vi "C-726.1CD (Piezo).vi"(8 "error in":errorcluster, 11 "System no.":i32=1 min=1 max=4 step=1) -> (0 "error out":errorcluster, 2 "Conn. Axis":string[](array[string]), 3 "C-726.1CD":dbl[](array[numeric]) format="%.6f", 5 "Identification 2":string)   [LabVIEW 2011]
panel:
  in  "stop":bool
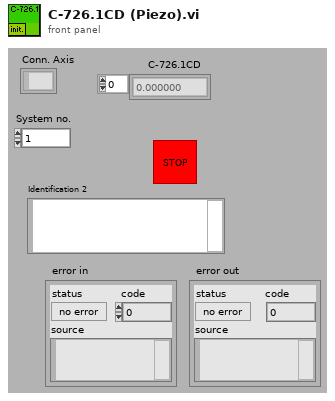
[diagram p1: front panel]
types:
  T1 = cluster{"Host address/name":string, "Port":i32, "Board":i32, "TCP/IP Search?":bool}
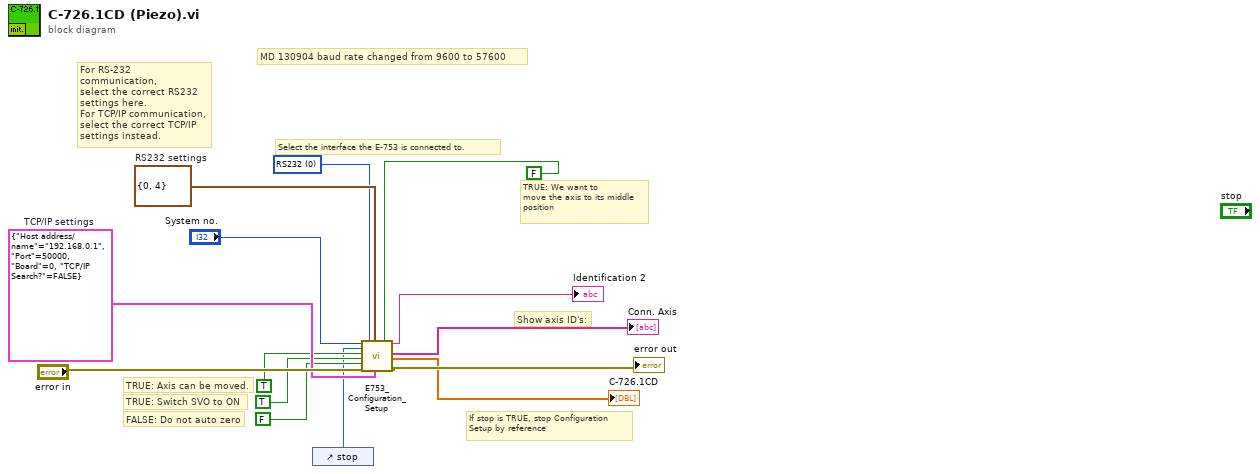
[diagram p0: block diagram]
diagram:
  w10 = cluster{"Portnumber":i32, "Baudrate":u16} {"Portnumber"=0, "Baudrate"=4}  # RS232 settings
  w11 = T1 {"Host address/name"="192.168.0.1", "Port"=50000, "Board"=0, "TCP/IP Search?"=FALSE}  # TCP/IP settings
  w8 = u16 0 items=["RS232", "TCP/IP"] ("Interface")
  # "MD 130904 baud rate changed from 9600 to 57600"
  # "TRUE: We want to\nmove the axis to its middle\nposition"
  # "FALSE: Do not auto zero"
  # "TRUE: Switch SVO to ON"
  # "If stop is TRUE, stop Configuration\nSetup by reference"
  # "For RS-232 communication,\nselect the correct RS232\nsettings here.\nFor TCP/IP communication, \nselect the correct TCP/IP\nsettings instead."
  # "Select the interface the E-753 is connected to."
  # "Show axis ID's:"
  # "TRUE: Axis can be moved."
  n1 = control-ref of="stop"() -> (w1:refnum<vi>)
  n2 = call "E753_Configuration_Setup.vi"("System no."="System no.", "Stop refnum"=w1, "Connected?"=TRUE ("All axes?"), "Change servo status to ON?"=TRUE ("Use dialog to define\nconnected stages?"), "Perform autozero?"=FALSE ("Use dialog to define\nconnected stages?"), "error in"="error in", "Interface"=w8, "RS232 settings"=w10, "TCP/IP settings"=w11, "Move to middle?"=FALSE ("Use dialog to define\nconnected stages?")) -> ("Identification"=→"Identification 2":string, "Conn. \nAxis"=→"Conn. Axis":string[], "Position"=→"C-726.1CD":dbl[], "error out"=→"error out":errorcluster)  [unwired: 3 in, 3 out]
